vi "POSTRequest.vi"(7 "Body in":string, 8 "error in (no error)":errorcluster, 9 "Parameter":string, 10 "Request":string, 11 "ByteRESTBase in":refnum<class "ByteRESTBase.lvclass">) -> (0 "error out":errorcluster, 1 "Headers":string, 2 "Body":string, 3 "ByteRESTBase out":refnum<class "ByteRESTBase.lvclass">)   [LabVIEW 2019, in "ByteREST.lvlib" / "ByteRESTBase.lvclass"]
doc: "Effettua una richiesta di GET al server come:\nSERVER/api/bytegs/RICHIESTA/PARAMETRO(opzionale)"
uses:
  ByteRESTBase.lvclass
  Status_Code.ctl
  ByteRESTBase.lvclass/ByteRESTBase.ctl
  <vilib>/httpClient/POSTBuffer.vi
  <vilib>/httpClient/LabVIEWHTTPClient.lvlib
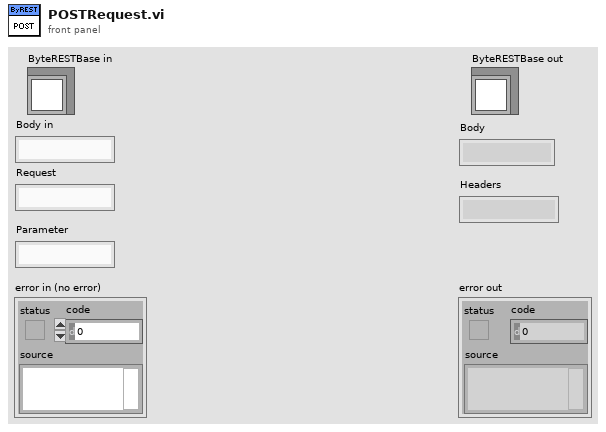
[diagram p1: front panel]
types:
  T1 = typedef "ByteREST.lvlib/ByteRESTBase.lvclass/Status_Code.ctl" = u16
  T2 = typedef "LabVIEWHTTPClient.lvlib/ClientHandle.ctl" = refnum<k1>
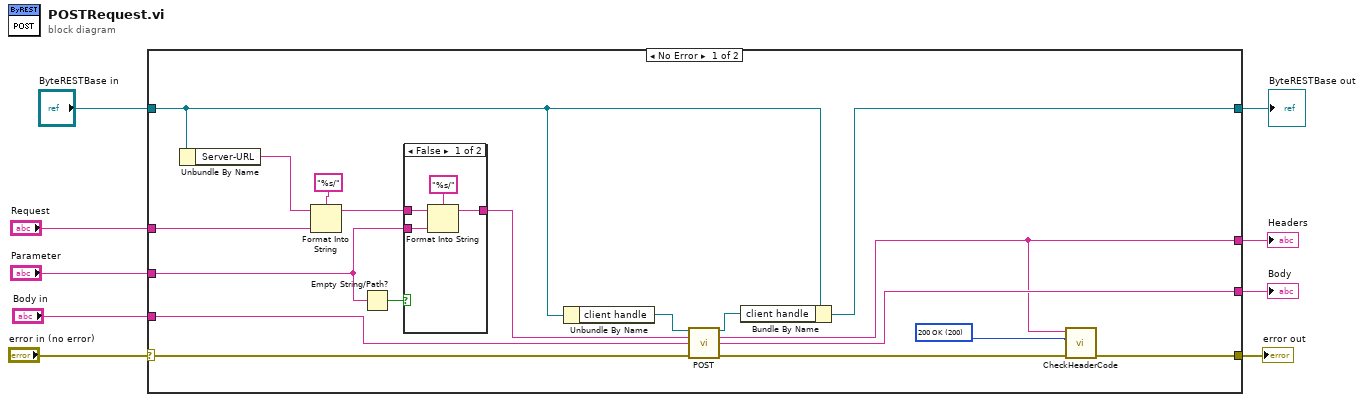
[diagram p0: block diagram]
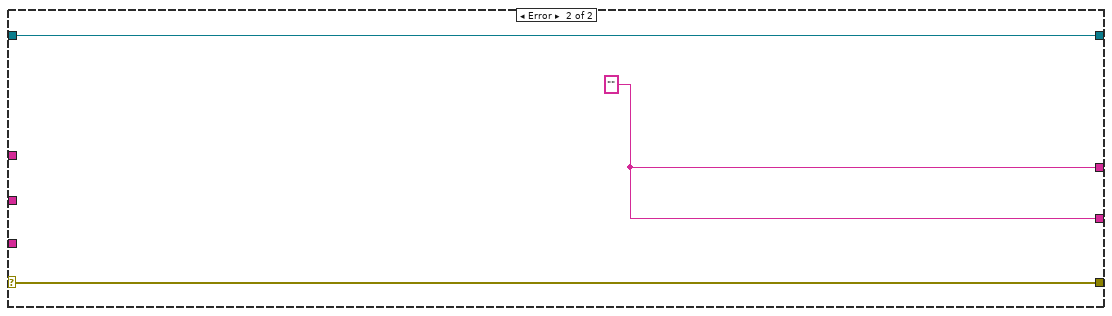
[diagram p3: hidden frame]
diagram:
  n1 = case shown="No Error" "error in (no error)" {
    selector: "error in (no error)" -> [w23 w35]
    tunnel: [w11 w35] -> w8
    tunnel: [w20 w34] -> w2
    tunnel: "ByteRESTBase in" -> [w17 w34]
    tunnel: "Request" -> [w15 _]
    tunnel: "Parameter" -> [w24 _]
    tunnel: [w19 w33] -> w5
    tunnel: [w12 w33] -> w4
    tunnel: "Body in" -> [w10 _]
    frame No Error {
      w13 = T1 200 items=["200 OK"=200, "201 Created"=201, "400 Bad Request"=400, "401 Unauthorized"=401, "403 Forbidden"=403, "404 Not Found"=404, "405 Method Not Allowed"=405, "406 Not Acceptable"=406, "500 Internal Server Error"=500] ("Code")
      n2 = Unbundle By Name(w17) -> ("Server-URL"=w16:string)
      n3 = Format Into String(format string="%s/" ("url"), initial string=w16, w15) -> (resulting string=w26:string)  [unwired: 1 in, 1 out]
      n4 = Empty String/Path?(string/path=w24) -> (empty?=w25:bool)
      n5 = case shown="False" w25 {
        tunnel: w26 -> [w30 w32]
        tunnel: [w28 w32] -> w22
        tunnel: w24 -> [w29 _]
        frame False {
          n6 = Format Into String(format string="%s/" ("url"), initial string=w30, w29) -> (resulting string=w28:string)  [unwired: 1 in, 1 out]
        }
        frame True {
        }
      }
      n7 = Unbundle By Name(w17) -> ("client handle"=w21:T2)
      n8 = call-poly <vilib>:"POST.vi"("client handle"=w21, "url"=w22, "buffer"=w10, "error in (no error)"=w23) -> ("client handle out"=w18:T2, "headers"=w12:string, "body"=w19:string, "error out"=w14:errorcluster)  [unwired: 8 in]
      n9 = Bundle By Name(cluster=w17, "client handle"=w18) -> (w20:refnum<class "ByteRESTBase.lvclass">)
      n10 = call "CheckHeaderCode.vi"("error in (no error)"=w14, "Expected code (200)"=w13, "Headers"=w12) -> ("error out"=w11:errorcluster)  [unwired: 8 in]
    }
    frame Error {
      w33 = "" ("body")
    }
  }
  "error out" <- w8
  "Body" <- w5
  "Headers" <- w4
  "ByteRESTBase out" <- w2
